vi "查询报警记录.vi"(6 "设备名":string, 8 "错误输入":errorcluster, 9 "大日期":string, 10 "小日期":string, 11 "数据库连接引用 i":T1) -> (0 "error out":errorcluster, 1 "累计剂量列":dbl[](array[numeric]), 2 "查询结果":string[][](array[string]), 3 "数据库连接引用 o":T1)   [LabVIEW 2016]
uses:
  <vilib>/addons/database/Connection.llb/Conn ObjectReference.ctl
  <vilib>/addons/database/NI_Database_API.lvlib
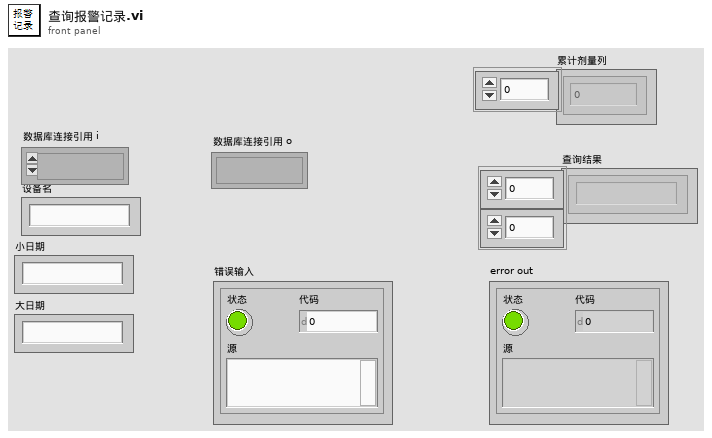
[diagram p1: front panel]
types:
  T1 = typedef "NI_Database_API.lvlib/Conn ObjectReference.ctl" = refnum<k1>
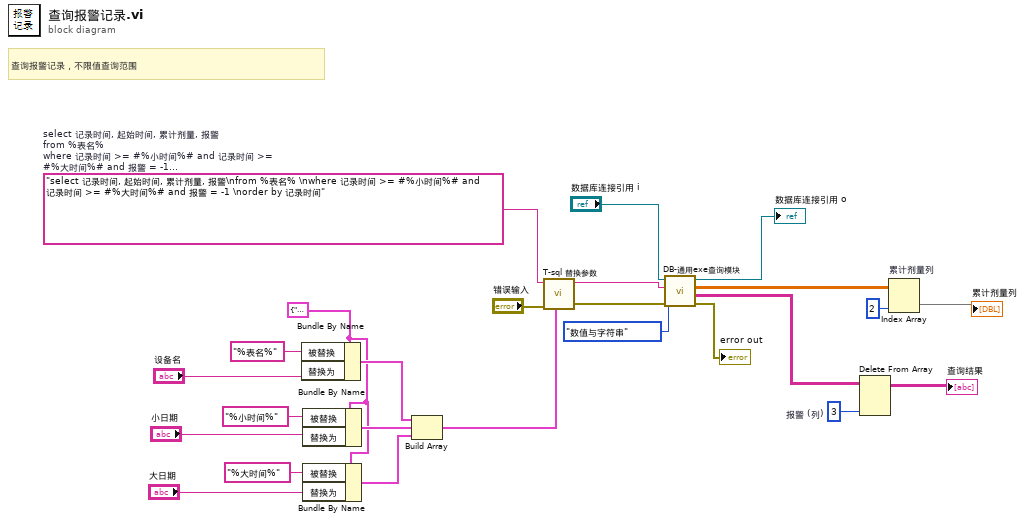
[diagram p0: block diagram]
diagram:
  w2 = 3  # 报警 (列)
  w5 = cluster{"被替换":string, "替换为":string} {"被替换"="", "替换为"=""} ("替换单元")
  w4 = "select 记录时间, 起始时间, 累计剂量, 报警\nfrom %表名% \nwhere 记录时间 >= #%小时间%# and 记录时间 >= #%大时间%# and 报警 = -1 \norder by 记录时间"  # select 记录时间, 起始时间, 累计剂量, 报警 from %表名%  where 记录时间 >= #%小时间%# and 记录时间 >= #%大时间%# and 报警 = -1  order by 记录时间
  # "查询报警记录，不限值查询范围"
  n1 = Bundle By Name(cluster=w5, "被替换"="%表名%", "替换为"="设备名") -> (w12:cluster{"被替换":string, "替换为":string})
  n2 = Bundle By Name(cluster=w5, "被替换"="%小时间%", "替换为"="小日期") -> (w13:cluster{"被替换":string, "替换为":string})
  n3 = Bundle By Name(cluster=w5, "被替换"="%大时间%", "替换为"="大日期") -> (w14:cluster{"被替换":string, "替换为":string})
  n4 = Build Array(w12, w13, w14) -> (w15:cluster{"被替换":string, "替换为":string}[])
  n5 = call "T-sql 替换参数.vi"("替换项"=w15, "错误输入"="错误输入", "T-sql 模板"=w4) -> ("错误输出"=w19:errorcluster, "T-sql"=w16:string)  [unwired: 7 in]
  n6 = call "DB-通用exe查询模块.vi"("error in (no error)"=w19, "解析模式"=enum16{"仅数值", "仅字符串", "数值与字符串"}."数值与字符串", "SQL query"=w16, "数据库连接引用"="数据库连接引用 i") -> ("error out"=→"error out":errorcluster, "字符串数据"=w3:string[][], "数值数据"=w23:dbl[][], "数据库连接引用out"=→"数据库连接引用 o":T1)  [unwired: 3 in, 1 out]
  n7 = Delete From Array(array=w3, index (col)=w2) -> (array with subset deleted=→"查询结果":string[][])  [unwired: 2 in, 1 out]
  n8 = Index Array "累计剂量列"(array=w23, index (col)=2 ("禁用的索引 (列)")) -> (element=→"累计剂量列":dbl[])  [unwired: 1 in]
